vi "sendMessage.vi"(8 "error in (no error)":errorcluster, 10 "message":string, 11 "TCPComEvents in":refnum<class "TCPComEvents.lvclass">) -> (0 "error out":errorcluster, 3 "TCPComEvents out":refnum<class "TCPComEvents.lvclass">)   [LabVIEW 2016, in "TCPComEvents.lvclass"]
uses:
  TCPComEvents.lvclass
  TCPComEvents.lvclass/TCPComEvents.ctl
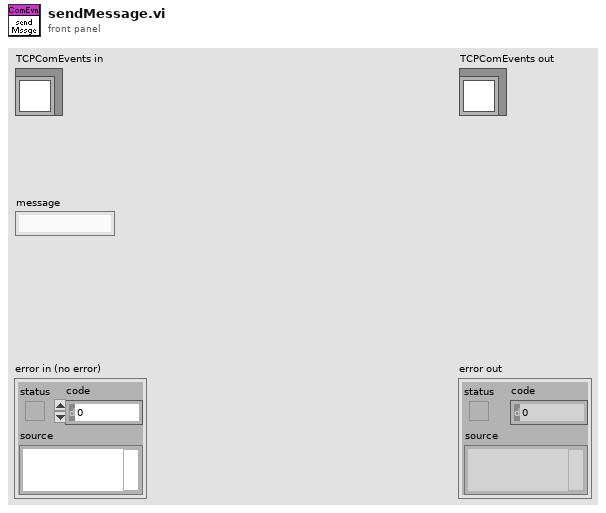
[diagram p1: front panel]
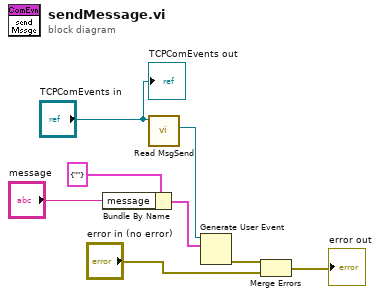
[diagram p0: block diagram]
diagram:
  n1 = Bundle By Name(cluster=cluster{"message":string} {"message"=""} ("event data"), "message"="message") -> (w5:cluster{"message":string})
  n2 = call "Read MsgSend.vi"("TCPComEvents in"="TCPComEvents in") -> ("MsgSend"=w4:refnum<user-event>)  [unwired: 8 in, 2 out]
  n3 = Generate User Event(user event=w4, event data cluster=w5) -> (error out=w2:errorcluster)  [unwired: 2 in, 1 out]
  n4 = Merge Errors(w2, "error in (no error)") -> (→"error out":errorcluster)
  "TCPComEvents out" <- "TCPComEvents in"
